vi "tag bus type to eip type.vi"(11 "data type":T1) -> (2 "valid?":bool, 3 "eip tag types":T2)   [LabVIEW 2013, in "EIP Tags Configuration.lvclass"]
uses:
  EIP Tags Configuration.lvclass
  eip tag types.ctl
  <vilib>/NI/Tag Bus/tag/Data Type.ctl
  <vilib>/NI/Tag Bus/tag/tag descriptor.lvclass
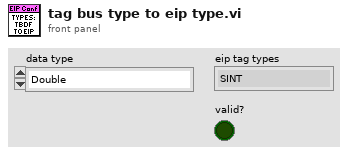
[diagram p1: front panel]
types:
  T1 = typedef "tag bus.lvlib/tag descriptor.lvclass/Data Type.ctl" = enum16{"Double", "Single", "I64", "I32", "I16", "I8", "U64", "U32", "U16", "U8", "Boolean", "String", "Array of Double", "Array of Single", "Array of I64", "Array of I32", "Array of I16", "Array of I8", "Array of U64", "Array of U32", "Array of U16", "Array of U8", "Array of Boolean", "Array of String"}
  T2 = typedef "EIP Tags Configuration.lvclass/eip tag types.ctl" = enum16{"SINT", "INT", "DINT", "REAL", "BOOL", "STRING"}
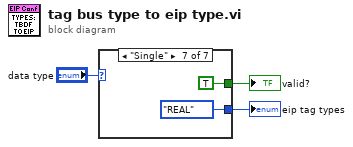
[diagram p0: block diagram]
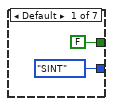
[diagram p2: hidden frame]
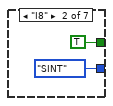
[diagram p3: hidden frame]
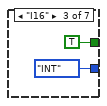
[diagram p4: hidden frame]
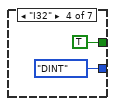
[diagram p5: hidden frame]
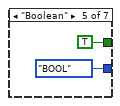
[diagram p6: hidden frame]
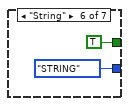
[diagram p7: hidden frame]
diagram:
  n1 = case shown="\"Single\"" "data type" {
    tunnel: [eip_tag_types."SINT" ("eip tag types") eip_tag_types."SINT" ("eip tag types") eip_tag_types."INT" ("eip tag types") eip_tag_types."DINT" ("eip tag types") eip_tag_types."BOOL" ("eip tag types") eip_tag_types."STRING" ("eip tag types") eip_tag_types."REAL" ("eip tag types")] -> w1
    tunnel: [FALSE TRUE TRUE TRUE TRUE TRUE TRUE] -> w2
    frame Default {
    }
    frame "I8" {
    }
    frame "I16" {
    }
    frame "I32" {
    }
    frame "Boolean" {
    }
    frame "String" {
    }
    frame "Single" {
    }
  }
  "eip tag types" <- w1
  "valid?" <- w2
